vi "getState.vi"(8 "error in (no error)":errorcluster, 11 "Originator in":refnum<class "Originator.lvclass">) -> (0 "error out":errorcluster, 2 "State":string, 3 "Originator out":refnum<class "Originator.lvclass">)   [LabVIEW 2018, in "Originator.lvclass"]
uses:
  Originator.lvclass
  Originator.lvclass/Originator.ctl
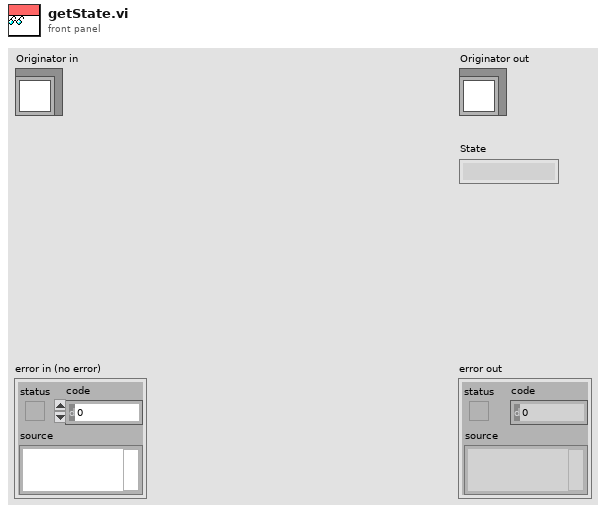
[diagram p1: front panel]
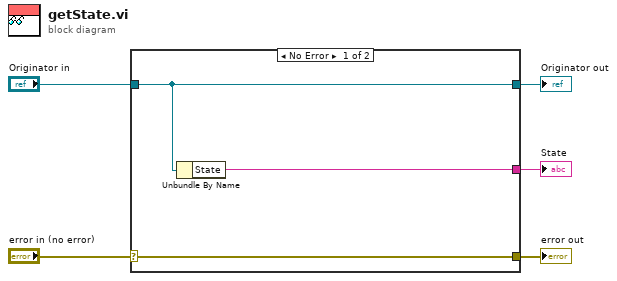
[diagram p0: block diagram]
diagram:
  n1 = case shown="No Error" "error in (no error)" {
    selector: "error in (no error)" -> [w8 w9]
    tunnel: [w8 w9] -> w4
    tunnel: [w7 w10] -> w2
    tunnel: "Originator in" -> [w7 w10]
    tunnel: [w6 _] -> w1
    frame No Error {
      n2 = Unbundle By Name(w7) -> ("State"=w6:string)
    }
    frame Error {
    }
  }
  "error out" <- w4
  "Originator out" <- w2
  "State" <- w1
